vi "B-Field - Bug1 Workaround.vi"(1 "Array 2":dbl[](array[numeric])) -> (0 "Array":dbl[](array[numeric]))   [LabVIEW 2009]
panel:
  # "This VI should not need to exist.  It gives a workaround for the fact that \nan acquisition refuses to run if it has an odd number of samples to \nacquire or generate\n\nErrro 600293"
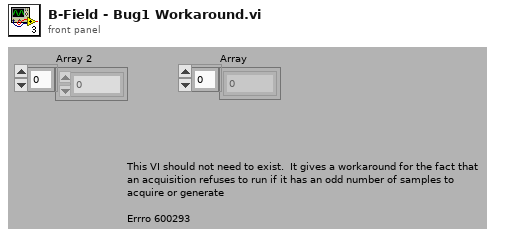
[diagram p1: front panel]
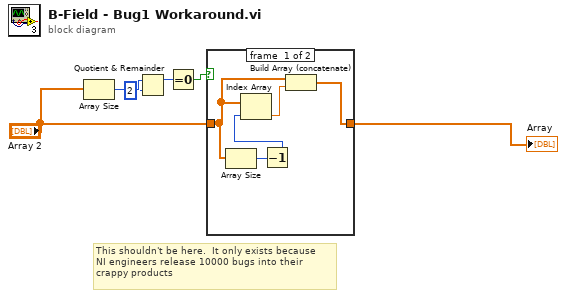
[diagram p0: block diagram]
diagram:
  # "This shouldn't be here.  It only exists because \nNI engineers release 10000 bugs into their \ncrappy products"
  n1 = Array Size(array="Array 2") -> (size(s)=w3:i32)
  n2 = Quotient & Remainder(x=w3, y=2) -> (x-y*floor(x/y)=w1:i32)  [unwired: 1 out]
  n3 = Equal To 0?(x=w1) -> (x = 0?=w4:bool)
  n4 = case shown="False" w4 {
    tunnel: "Array 2" -> [w11 w12]
    tunnel: [w9 w12] -> w6
    frame #0 {
      n5 = Array Size(array=w11) -> (size(s)=w8:i32)
      n6 = Decrement(x=w8) -> (x-1=w7:i32)
      n7 = Index Array(array=w11, index=w7) -> (element=w10:dbl)
      n8 = Build Array (concatenate)(w11, w10) -> (w9:dbl[])
    }
    frame #1 {
    }
  }
  "Array" <- w6
